vi "Test Abs Boolean.vi"(4 "Abs_Boolean.lvclass":refnum<class "Abs_Boolean.lvclass">) -> (1 "abs_Node":refnum<class "bt_Node.lvclass">)   [LabVIEW 2021, in "BT.lvlib"]
uses:
  BT.lvlib
  Support/Nodes/abs_Node/bt_Node.lvclass
  <vilib>/TSA/Abstract Data Classes/Abs_Types/Boolean/Abs_Boolean.lvclass
  C:/Program Files (x86)/National Instruments/LabVIEW 2021/vi.lib/TSA/Abstract Data Classes/Abs_Types/Type/Abs_Type.lvclass
  Support/Nodes/Leaves/Test Boolean/Test Abs_Boolean.lvclass
  C:/Users/Tim/Documents/GitHub/LV_Behaviour_Tree/BT Abstract Type/abs_Type Leaf/abs_Type Leaf.lvclass
  C:/Users/Tim/Documents/GitHub/LV_Behaviour_Tree/Source/Support/Nodes/abs_Node/bt_Node.lvclass
  Support/Nodes/Leaves/abs_Type Leaf/abs_Type Leaf.lvclass/abs_Type Leaf.ctl
  Support/Nodes/Leaves/abs_Type Leaf/Properties/Write Value Class.vi
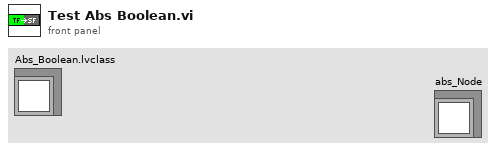
[diagram p1: front panel]
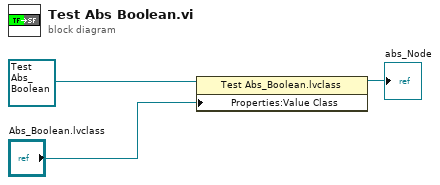
[diagram p0: block diagram]
diagram:
  n1 = property class="Test Abs_Boolean.lvclass"(reference=refnum<class "Test Abs_Boolean.lvclass"> refnum ("BT.lvlib:Test Boolean.lvclass"), "Properties:Value Class"="Abs_Boolean.lvclass") -> (reference out=→"abs_Node":refnum<class "Test Abs_Boolean.lvclass">)  [unwired: 1 in, 1 out]
